vi "PID_tuningPacket.vi"(9 "Float Array":sgl[](array[numeric]), 10 "Automatic":u8) -> (2 "string":string, 3 "Byte Array":u8[](array[numeric]) format="%x")   [LabVIEW 2014]
panel:
  # "0xb6 0xf3 0x9d 0x3f"
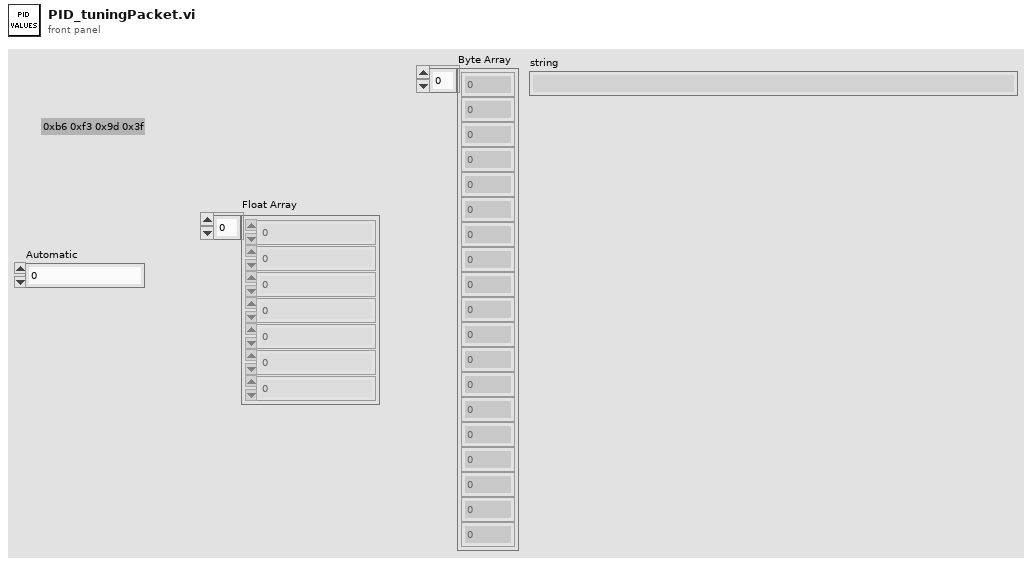
[diagram p1: front panel]
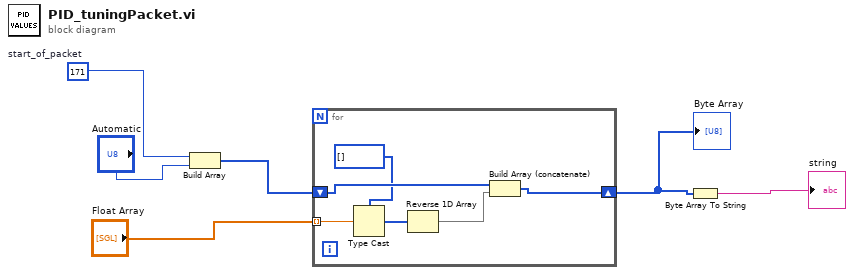
[diagram p0: block diagram]
diagram:
  w1 = u8 171  # start_of_packet
  n1 = Build Array(w1, "Automatic") -> (w4:u8[])
  n2 = for {
    tunnel: "Float Array" -> [w12] mode=indexing
    shift-right: [w7] -> w3
    shift-left: w4 -> [w11]
    n3 = Type Cast(type=u8[] [], x=w12) -> (*(type *) &x=w9:u8[])
    n4 = Reverse 1D Array(array=w9) -> (reversed array=w8:u8[])
    n5 = Build Array (concatenate)(w11, w8) -> (w7:u8[])
  }
  "Byte Array" <- w3
  n6 = Byte Array To String(unsigned byte array=w3) -> (string=→"string":string)
